vi "Finish.vi"() -> ()   [LabVIEW 2016]
doc: "This VI is called just before exiting. It is expected to close I/O refnum, save collected data, etc."
uses:
  Refname/Queues.ctl
  Refname/Sensors.ctl
  Refname/Refname to String (Sensors).vi
panel:
  out "size(s)":i32
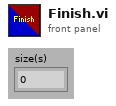
[diagram p1: front panel]
types:
  T1 = typedef "Sensors.ctl" = enum16{"DIP 1", "DIP 2", "DIP 3", "DIP 4", "IMU", "HuskieBoard"}
  T2 = typedef "Queues.ctl" = enum16{"Log Queue"}
  T3 = typedef "WPI_SerialPortRef.ctl" = cluster{"DevStatus":errorcluster, "Serial Port Name":refnum<visa-resource-name>}
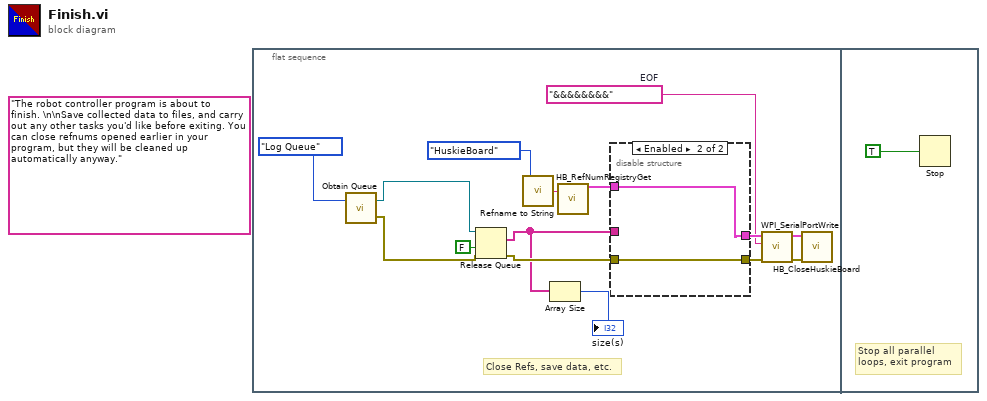
[diagram p0: block diagram]
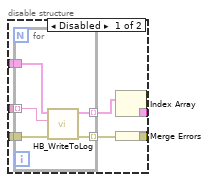
[diagram p2: hidden frame]
diagram:
  (unwired) "The robot controller program is about to finish. \n\nSave collected data to files, and carry out any other tasks you'd like before exiting. You can close refnums opened earlier in your program, but they will be cleaned up automatically anyway."
  n1 = flat-sequence {
    frame #0 {
      w1 = "&&&&&&&&"  # EOF
      # "Close Refs, save data, etc."
      n2 = call "Obtain Queue.vi"("Queue"=Queues."Log Queue") -> ("error out"=w12:errorcluster, "Queue Ref"=w11:refnum<queue>)  [unwired: 1 in]
      n3 = Release Queue(queue=w11, force destroy? (F)=FALSE, error in (no error)=w12) -> (remaining elements=w7:string[], error out=w13:errorcluster)  [unwired: 1 out]
      n4 = call-poly "Refname to String.vi"("Enum"=Sensors."HuskieBoard") -> ("String"=w9:string)
      n5 = Array Size(array=w7) -> (size(s)=→"size(s)":i32)
      n6 = call <vilib>:"HB_RefNumRegistryGet.vi"("refnum name"=w9) -> ("HBDevRef"=w8:T3)  [unwired: 13 in, 1 out]
      n7 = disable-structure shown="Enabled" {
        disable-tunnel: [w21 w29] -> w5
        disable-tunnel: [w19 w28] -> w4
        disable-tunnel: w13 -> [w18 w28]
        disable-tunnel: w8 -> [w17 w29]
        disable-tunnel: w7 -> [w16 _]
        frame Disabled {
          n8 = for {
            tunnel: w16 -> [w27] mode=indexing
            tunnel: [w26] -> w22 mode=indexing
            tunnel: w18 -> [w25]
            tunnel: [w24] -> w20 mode=indexing
            tunnel: w17 -> [w23]
            n9 = call <vilib>:"HB_WriteToLog.vi"("error in (no error)"=w25, "Log string"=w27, "HBDevRef"=w23) -> ("error out"=w24:errorcluster, "HBDevRef"=w26:T3)  [unwired: 7 in]
          }
          n10 = Index Array(array=w22) -> (element=w21:T3)  [unwired: 1 in]
          n11 = Merge Errors(w20) -> (w19:errorcluster)
        }
        frame Enabled {
        }
      }
      n12 = call <vilib>:"WPI_SerialPortWrite.vi"("error in (no error)"=w4, "Buffer"=w1, "SerialPortRef"=w5) -> ("error out"=w3:errorcluster, "SerialPortRef"=w2:T3)  [unwired: 6 in, 1 out]
      n13 = call <vilib>:"HB_CloseHuskieBoard.vi"("error in (no error)"=w3, "HBDeviceRef"=w2) -> ()  [unwired: 9 in, 1 out]
    }
    frame #1 {
      # "Stop all parallel\nloops, exit program"
      n14 = Stop(stop? (T)=TRUE ("Quit")) -> ()
    }
  }
